vi "multi ROI test.vi"() -> ()   [LabVIEW 2013]
doc: "This example shows how to compute the histogram of an image or a region in the image. This example also shows how to set up and use the display tools to select and work on different regions in the image interactively."
uses:
  <vilib>/vision/Image Controls.llb/IMAQ Image.ctl
  <vilib>/vision/NI_Vision_Development_Module.lvlib
panel:
  in  "添加按钮":bool
  out "Histogram 2":T1(graph)
  in  "Stop 2":bool
  out "Image":T2(plugin-control)
  # "Overview: Demonstrates how to use the IMAQ Histogram function with a mask to return histogram information about the portion of the image in a Region of Interest (ROI).\nRequirements: Vision Development Software.\nInstructions:\n1. Run the VI.\n2. Draw a ROI in the image by left clicking, hold left mouse button down, drag the mouse across the image, and release the mouse button."
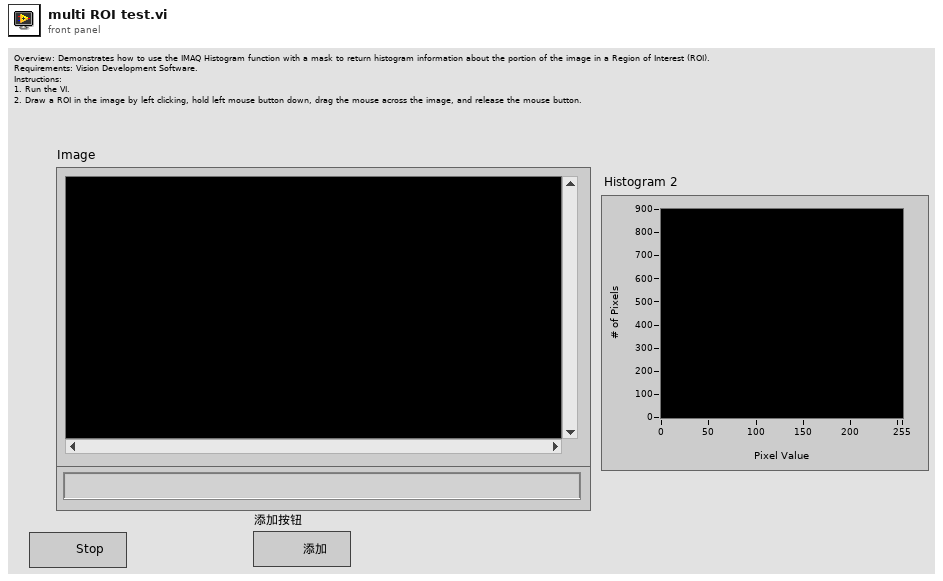
[diagram p1: front panel]
types:
  T1 = cluster{"Starting Value":sgl, "Incremental Value":sgl, "Histogram":u32[]}
  T2 = typedef "IMAQ Image.ctl" = refnum<image>
  T3 = typedef "IMAQ Rectangle" = cluster{"Left":i32, "Top":i32, "Right":i32, "Bottom":i32, "Rotation":dbl}
  T4 = typedef "ROI Descriptor" = cluster{"Global Rectangle":i32[], "Contours":cluster{"ID":enum32{"External", "Internal"}, "Type":u32, "Coordinates":i32[]}[]}
  T5 = cluster{"Global Rectangle":i32[], "Contours":cluster{"Contour Type":u32, "ROI Type":u32, "Points":i32[]}[]}
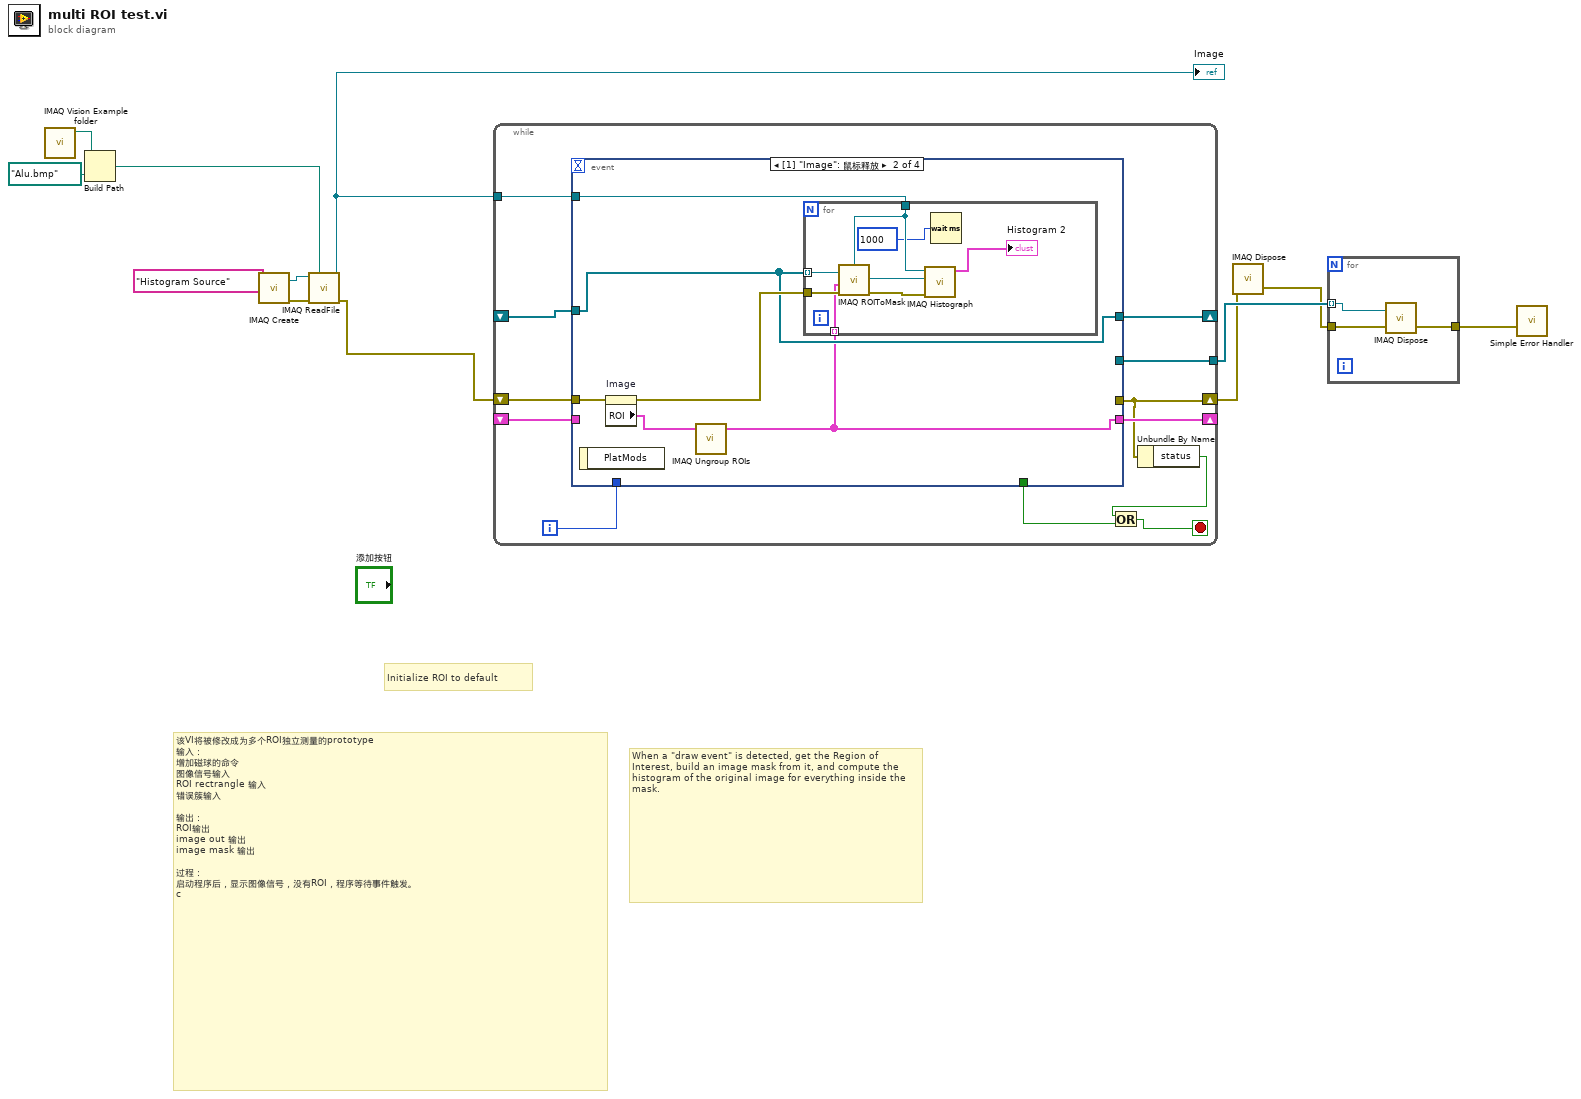
[diagram p0: block diagram]
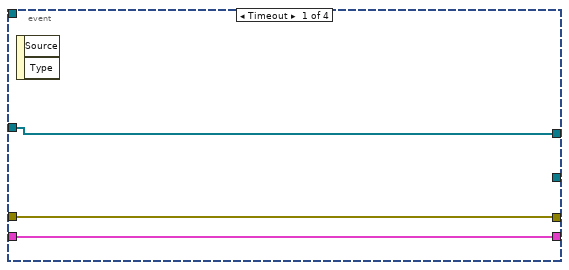
[diagram p2: hidden frame]
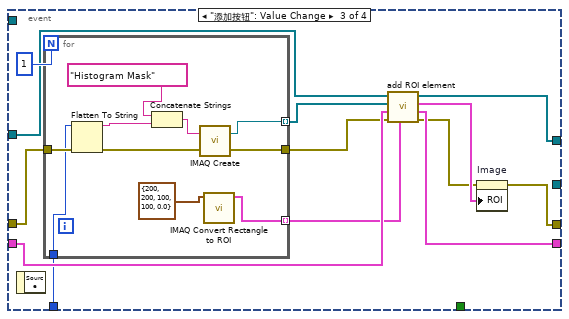
[diagram p3: hidden frame]
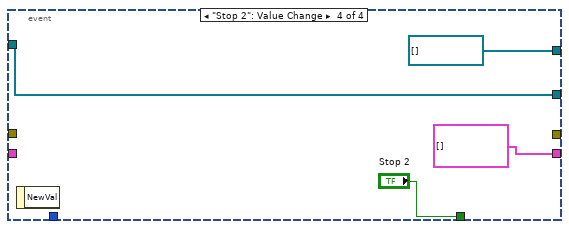
[diagram p4: hidden frame]
diagram:
  # "该VI将被修改成为多个ROI独立测量的prototype\n输入：\n增加磁球的命令\n图像信号输入\nROI rectrangle 输入\n错误簇输入\n\n输出：\nROI输出\nimage out 输出\nimage mask 输出\n\n过程：\n启动程序后，显示图像信号，没有ROI，程序等待事件触发。\nc"
  # "Initialize ROI to default"
  # "When a \"draw event\" is detected, get the Region of Interest, build an image mask from it, and compute the histogram of the original image for everything inside the mask."
  n1 = call "IMAQ Vision Example folder.vi"() -> ("Example Image Path"=w12:path)  [unwired: 11 in]
  n2 = Build Path(base path=w12, name or relative path=path "Alu.bmp") -> (appended path=w6:path)
  n3 = call "IMAQ Create"("Image Name"="Histogram Source") -> ("New Image"=w11:T2, "error out"=w10:errorcluster)  [unwired: 4 in]
  n4 = call "IMAQ ReadFile"("File Path"=w6, "error in (no error)"=w10, "Image"=w11) -> ("error out"=w1:errorcluster, "Image Out"=w8:T2)  [unwired: 4 in, 3 out]
  "Image" <- w8
  n5 = while {
    tunnel: [w23] -> w5
    tunnel: w8 -> [w22]
    shift-right: [w18] -> _
    shift-left: _ -> [w19]
    shift-right: [w17] -> _
    shift-left: _ -> [w16]
    shift-right: [w15] -> w2
    shift-left: w1 -> [w24]
    i -> [w13]
    stop <- w20 stop-if-true
    n6 = event shown="[1] \"Image\": 鼠标释放" {
      selector: _ -> [_ _ _ _]
      dyn-events: _ -> [_ _ _ _]
      timeout: _ -> [_ _ _ _]
      tunnel: [_ _ _ w67] -> w23
      tunnel: w24 -> [w25 w32 w52 _]
      tunnel: w22 -> [_ w33 _ _]
      tunnel: [w25 _ w46 _] -> w15
      tunnel: [_ _ _ "Stop 2"] -> w21
      tunnel: w19 -> [w27 w29 w45 w67]
      tunnel: [w27 w29 w53 T2[] []] -> w18
      tunnel: [w26 w28 w50 T4[] [] ("image ROI out")] -> w17
      tunnel: w16 -> [w26 _ w51 _]
      tunnel: w13 -> [_ _ w42 _]
      event Timeout {
        n7 = event-data() -> ()  [unwired: 1 in, 2 out]
      }
      event "Image": Mouse Up {
        n8 = event-data() -> ()  [unwired: 1 in, 1 out]
        n9 = property on="Image" class="ImageControl"(error in=w32) -> (error out=w31:errorcluster, "ROI"=w30:T5)  [unwired: 1 in, 1 out]
        n10 = call "IMAQ Ungroup ROIs"("ROI Descriptor"=w30) -> ("ROI Descriptors out"=w28:T4[])  [unwired: 3 in, 1 out]
        n11 = for {
          tunnel: w33 -> [w41]
          tunnel: w31 -> [w37]
          tunnel: w29 -> [w36] mode=indexing
          tunnel: w28 -> [w35] mode=indexing
          n12 = call "IMAQ ROIToMask"("error in (no error)"=w37, "ROI Descriptor"=w35, "Image"=w36, "Image Model"=w41) -> ("error out"=w39:errorcluster, "Image Out"=w40:T2)  [unwired: 2 in, 1 out]
          n13 = call "IMAQ Histograph"("error in (no error)"=w39, "Image Mask"=w40, "Image"=w41) -> ("Histogram Graph"=→"Histogram 2":T1)  [unwired: 5 in, 3 out]
          n14 = Wait (ms)(milliseconds to wait=u32 1000 ("毫秒计时值")) -> ()  [unwired: 1 out]
        }
      }
      event "添加按钮": Value Change {
        n15 = event-data() -> ()  [unwired: 1 in, 1 out]
        n16 = for {
          N: 1 -> [_]
          tunnel: [w61] -> w49
          tunnel: w52 -> [w60]
          tunnel: [w59] -> w44 mode=indexing
          tunnel: [w57] -> w43 mode=indexing
          tunnel: w42 -> [w55]
          n17 = Flatten To String(anything=w55, error in (no error)=w60) -> (data string=w63:string, error out=w56:errorcluster)  [unwired: 2 in, 1 out]
          n18 = Concatenate Strings("Histogram Mask" ("Image Name"), w63) -> (w62:string)
          n19 = call "IMAQ Create"("Image Name"=w62, "error in (no error)"=w56) -> ("New Image"=w59:T2, "error out"=w61:errorcluster)  [unwired: 3 in]
          n20 = call "IMAQ Convert Rectangle to ROI"("Rectangle"=T3 {"Left"=200, "Top"=200, "Right"=100, "Bottom"=100, "Rotation"=0.0} ("Default Rectangle")) -> ("ROI Descriptor"=w57:T4)  [unwired: 8 in, 1 out]
        }
        n21 = call "add ROI element.vi"("new ROI in"=w43, "错误输入（无错误）"=w49, "image ROI in"=w51, "new mask in"=w44, "image mask  in"=w45) -> ("错误输出"=w47:errorcluster, "image ROI out"=w50:T4[], "ROI Descriptor out"=w48:T4, "image mask out"=w53:T2[])  [unwired: 3 in]
        n22 = property on="Image" class="ImageControl"(error in=w47, "ROI"=w48) -> (error out=w46:errorcluster)  [unwired: 1 in, 1 out]
      }
      event "Stop 2": Value Change {
        n23 = event-data() -> ()  [unwired: 1 in, 1 out]
      }
    }
    n24 = Unbundle By Name(w15) -> ("status"=w14:bool)
    n25 = Or(x=w14, y=w21) -> (x .or. y?=w20:bool)
  }
  n26 = call "IMAQ Dispose"("error in (no error)"=w2) -> ("error out"=w4:errorcluster)  [unwired: 5 in]
  n27 = for {
    tunnel: w5 -> [w71] mode=indexing
    tunnel: w4 -> [w70]
    tunnel: [w69] -> w3
    n28 = call "IMAQ Dispose"("Image"=w71, "error in (no error)"=w70) -> ("error out"=w69:errorcluster)  [unwired: 4 in]
  }
  n29 = call <vilib>:"Simple Error Handler.vi"("error in (no error)"=w3) -> ()  [unwired: 4 in, 5 out]
